vi "STDpH_获取温度和测量值.vi"(8 "error in (no error)":errorcluster caption="错误输入（无错误）", 11 "MB session in":refnum<class "MB_Master.lvclass">) -> (0 "error out":errorcluster caption="错误输出", 2 "STDpH":cluster{"温度测量值":sgl, "pH":sgl, "信号值":sgl}, 3 "MB session out":refnum<class "MB_Master.lvclass">)   [LabVIEW 2016, in "斯坦道多参数.lvlib"]
uses:
  <vilib>/Plasmionique/MB Master/MB_Master/MB_Master.lvclass
  <vilib>/Plasmionique/MB Master/MB Master.lvlib
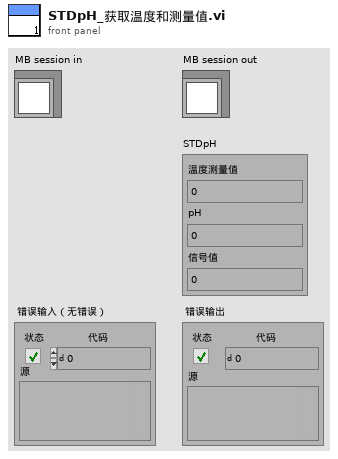
[diagram p1: front panel]
types:
  T1 = cluster{"pH":u32, "DO":u32, "Cond":u32, "Turb":u32, "叶绿素a":u32, "藻密度":u32, "ORP":u32, "COD":u32, "氯化物":u32, "氨氮":u32, "水中油":u32}
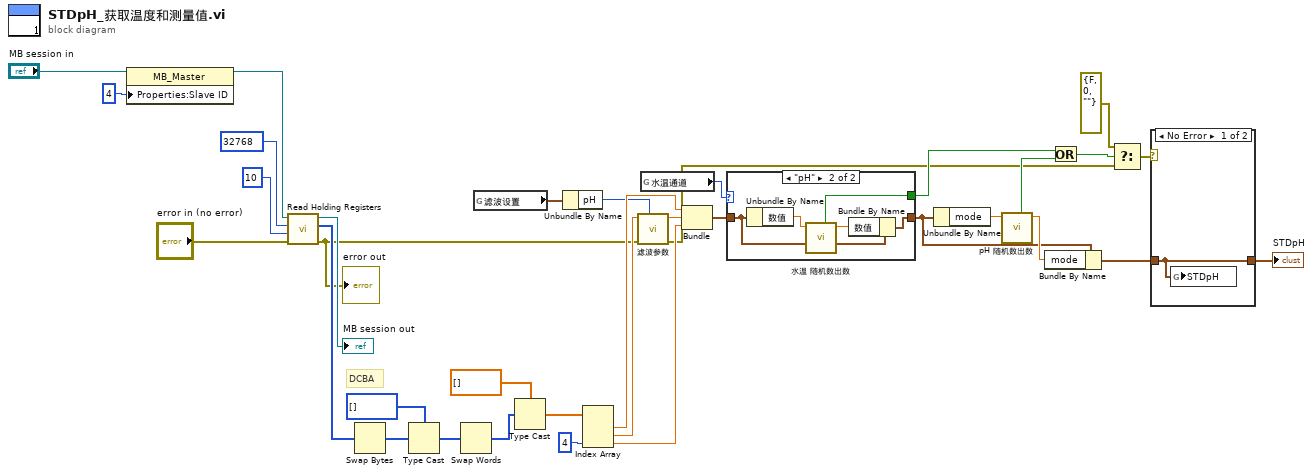
[diagram p0: block diagram]
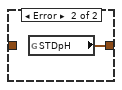
[diagram p3: hidden frame]
diagram:
  # "DCBA"
  n1 = property class="MB_Master"(reference="MB session in", "Properties:Slave ID"=u16 4 ("y")) -> (reference out=w20:refnum<class "MB_Master.lvclass">)  [unwired: 1 in, 1 out]
  n2 = call <vilib>:"Read Holding Registers.vi"("error in (no error)"="error in (no error)", "quantity"=u16 10, "starting address"=u16 32768, "MB session in"=w20) -> ("error out"=w3:errorcluster, "Registers"=w27:u16[], "MB session out"=→"MB session out":refnum<class "MB_Master.lvclass">)  [unwired: 5 in]
  "error out" <- w3
  n3 = Swap Bytes(anything=w27) -> (byte swapped=w26:u16[])
  n4 = Type Cast(type=u32[] [] ("数组 2"), x=w26) -> (*(type *) &x=w30:u32[])
  n5 = Swap Words(1:w30) -> (0:w32:u32[])
  n6 = global read "断电保存变量.vi" "滤波设置"() -> (w22:T1)
  n7 = Type Cast(type=sgl[] [] ("数组 2"), x=w32) -> (*(type *) &x=w18:sgl[])
  n8 = Unbundle By Name(w22) -> ("pH"=w21:u32)
  n9 = Index Array(array=w18, index #3=4 ("索引")) -> (element #1=w25:sgl, element #2=w17:sgl, element #3=w15:sgl)  [unwired: 2 in]
  n10 = call "滤波参数.vi"("滤波次数"=w21, "error in (no error)"=w3, "x"=w17) -> ("mode"=w16:dbl)  [unwired: 7 in, 1 out]
  n11 = global read "断电保存变量.vi" "水温通道"() -> (w11:enum16{"pH", "DO", "浊度", "电导率", "叶绿素a", "藻密度"})
  n12 = Bundle("数值"=w25, "mode"=w16, "数值"=w15) -> (w7:cluster{"数值":sgl, "mode":dbl, "数值":sgl})  [unwired: 1 in]
  n13 = case shown="\"pH\"" w11 {
    tunnel: w7 -> [w35 w39]
    tunnel: [w35 w37] -> w10
    tunnel: [_ w36] -> w5
    frame Default {
    }
    frame "pH" {
      n14 = Unbundle By Name(w39) -> ("数值"=w40:sgl)
      n15 = call "水温 随机数出数.vi"("原始值"=w40) -> ("取值输出"=w38:dbl, "x .and. y?"=w36:bool)  [unwired: 6 in, 1 out]
      n16 = Bundle By Name(cluster=w39, "数值"=w38) -> (w37:cluster{"数值":sgl, "mode":dbl, "数值":sgl})
    }
  }
  n17 = Unbundle By Name(w10) -> ("mode"=w13:dbl)
  n18 = call "pH 随机数出数.vi"("原始值"=w13) -> ("取值输出"=w12:dbl, "x .and. y?"=w6:bool)  [unwired: 6 in, 1 out]
  n19 = Bundle By Name(cluster=w10, "mode"=w12) -> (w8:cluster{"数值":sgl, "mode":dbl, "数值":sgl})
  n20 = Or(x=w5, y=w6) -> (x .or. y?=w4:bool)
  n21 = Select(t=errorcluster {"status"=FALSE, "code"=0, "source"=""}, s=w4, f=w3) -> (s? t:f=w1:errorcluster)
  n22 = case shown="No Error" w1 {
    tunnel: w8 -> [w41 _]
    tunnel: [w41 w42] -> w9
    frame No Error {
      n23 = global write "禹山过程全局变量.vi" "STDpH"(w41) -> ()
    }
    frame Error {
      n24 = global read "禹山过程全局变量.vi" "STDpH"() -> (w42:cluster{"温度测量值":sgl, "pH":sgl, "信号值":sgl})
    }
  }
  "STDpH" <- w9
